vi "Module Init.vi"(8 "error in (no error)":errorcluster, 11 "Hardware Info Module in":refnum<class "Hardware Info Module.lvclass">) -> (0 "error out":errorcluster, 3 "Hardware Info Module out":refnum<class "Hardware Info Module.lvclass">)   [LabVIEW 2020, in "Volatus.lvlib" / "Hardware Info Module.lvclass"]
uses:
  Hardware Info Module.lvclass
  Hardware Info Module.lvclass/Hardware Info Module.ctl
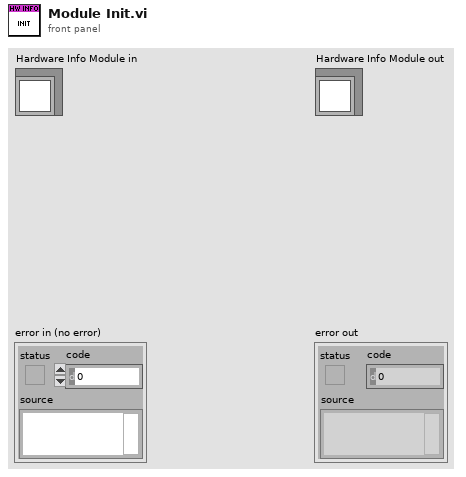
[diagram p1: front panel]
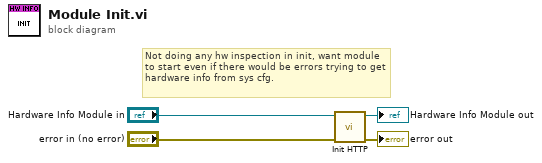
[diagram p0: block diagram]
diagram:
  # "Not doing any hw inspection in init, want module to start even if there would be errors trying to get hardware info from sys cfg."
  n1 = call "Init HTTP.vi"("error in (no error)"="error in (no error)", "Hardware Info Module in"="Hardware Info Module in") -> ("error out"=→"error out":errorcluster, "Hardware Info Module out"=→"Hardware Info Module out":refnum<class "Hardware Info Module.lvclass">)  [unwired: 8 in]
